vi "gentec-M-Link.Set Head Attenuator.vi"(0 "VISA resource In":refnum<visa-resource-name>, 2 "Set Head Attenuator":bool, 5 "error in (no error)":errorcluster) -> (11 "Data Read":string, 13 "Read Timeout":bool, 14 "VISA resource Out":refnum<visa-resource-name>, 16 "Max Lambda":i32, 17 "Min Lambda":i32, 19 "error out":errorcluster)   [LabVIEW 2014, in "gentec-M-Link - Driver.lvlib"]
doc: "Data to write: wat"
uses:
  gentec-M-Link - Driver.lvlib
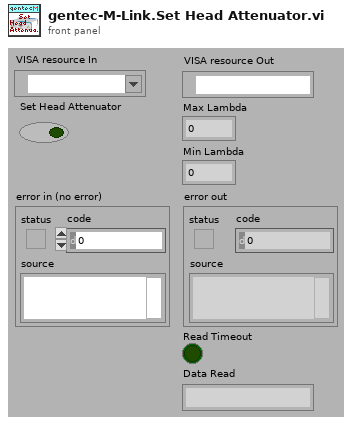
[diagram p1: front panel]
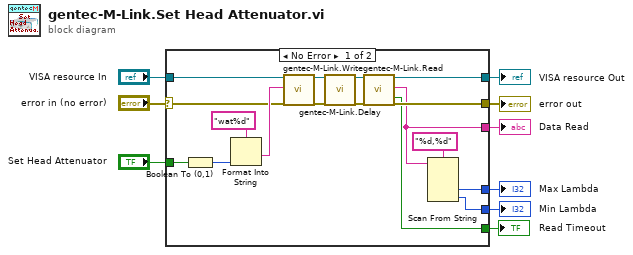
[diagram p0: block diagram]
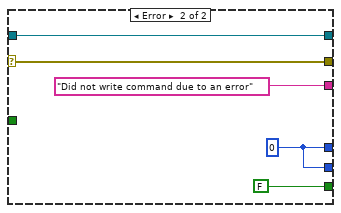
[diagram p2: hidden frame]
diagram:
  n1 = case shown="No Error" "error in (no error)" {
    selector: "error in (no error)" -> [w18 w31]
    tunnel: [w20 w31] -> w8
    tunnel: [w17 w28] -> w7
    tunnel: [w16 w28] -> w6
    tunnel: [w15 w30] -> w5
    tunnel: "VISA resource In" -> [w14 w30]
    tunnel: [w13 "Did not write command due to an error" ("Data Read")] -> w3
    tunnel: "Set Head Attenuator" -> [w12 _]
    tunnel: [w10 FALSE ("Read Timeout")] -> w1
    frame No Error {
      n2 = Boolean To (0,1)(Boolean=w12) -> (0, 1=w11:i16)
      n3 = Format Into String(format string="wat%d", w11) -> (resulting string=w25:string)  [unwired: 2 in, 1 out]
      n4 = call "gentec-M-Link.Write.vi"("VISA resource (In)"=w14, "Data To Write"=w25, "error in (no error)"=w18) -> ("VISA resource (Out)"=w24:refnum<visa-resource-name>, "error out"=w23:errorcluster)  [unwired: 14 in, 1 out]
      n5 = call "gentec-M-Link.Delay.vi"("VISA resource In"=w24, "error in (no error)"=w23) -> ("VISA resource Out"=w22:refnum<visa-resource-name>, "error out"=w21:errorcluster)  [unwired: 16 in]
      n6 = call "gentec-M-Link.Read.vi"("VISA resource (In)"=w22, "error in (no error)"=w21) -> ("VISA resource (Out)"=w15:refnum<visa-resource-name>, "Data Read"=w13:string, "Read Timeout"=w10:bool, "error out"=w20:errorcluster)  [unwired: 13 in, 1 out]
      n7 = Scan From String(format string="%d,%d", input string=w13) -> (output 1=w17:i32, output 2=w16:i32)  [unwired: 4 in, 3 out]
    }
    frame Error {
      w28 = 0
    }
  }
  "error out" <- w8
  "Max Lambda" <- w7
  "Min Lambda" <- w6
  "VISA resource Out" <- w5
  "Data Read" <- w3
  "Read Timeout" <- w1
